vi "Host - TCP Serial.vi"(8 "error in (no error)":errorcluster, 9 "port":u16=4001, 10 "address":string="192.168.81.105") -> ()   [LabVIEW 2021]
panel:
  out "x-y":u32
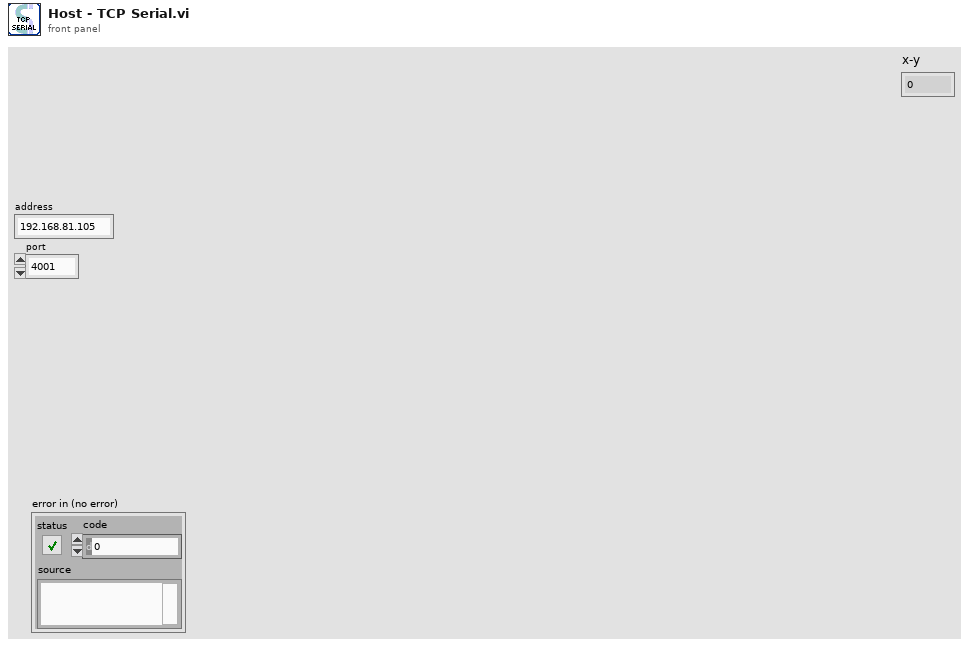
[diagram p1: front panel]
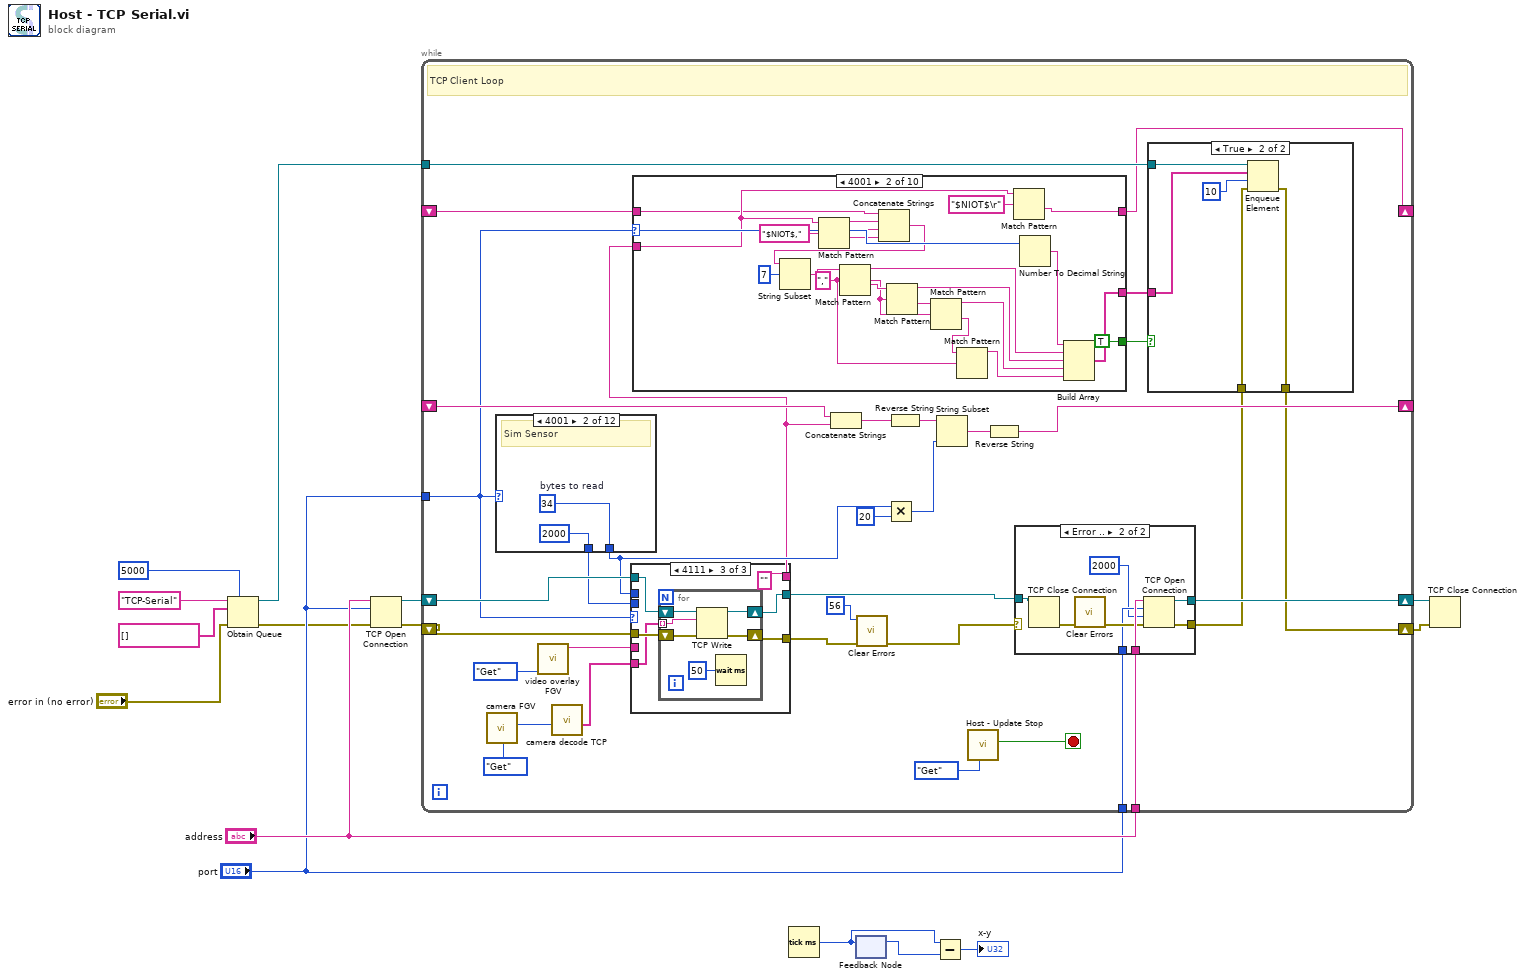
[diagram p0: block diagram]
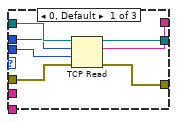
[diagram p3: hidden frame]
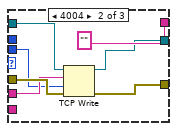
[diagram p4: hidden frame]
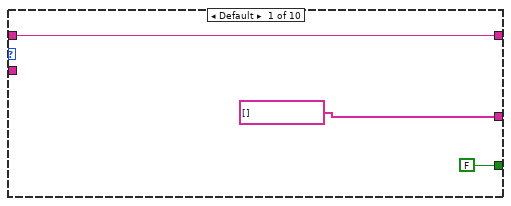
[diagram p5: hidden frame]
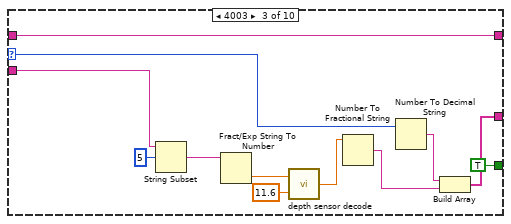
[diagram p6: hidden frame]
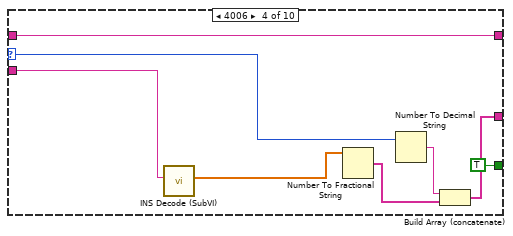
[diagram p7: hidden frame]
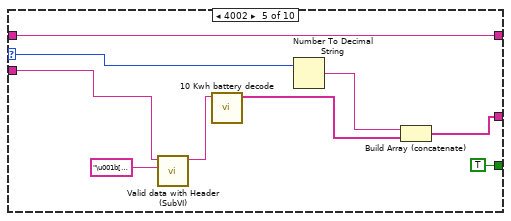
[diagram p8: hidden frame]
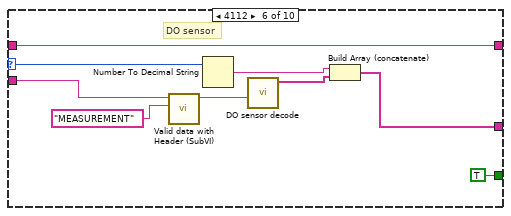
[diagram p9: hidden frame]
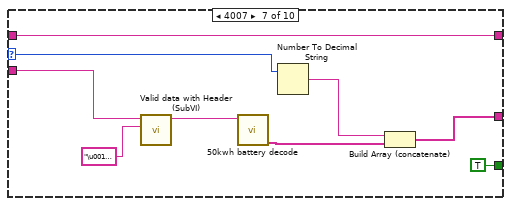
[diagram p10: hidden frame]
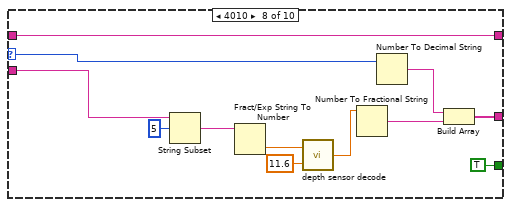
[diagram p11: hidden frame]
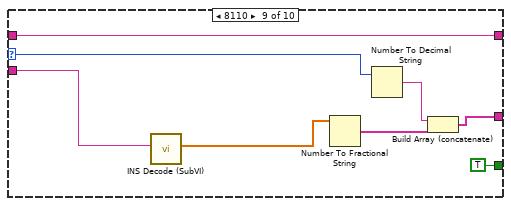
[diagram p12: hidden frame]
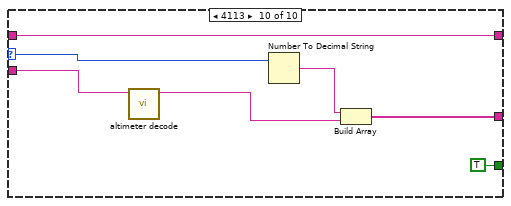
[diagram p13: hidden frame]
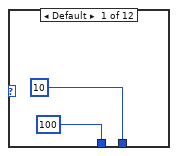
[diagram p15: hidden frame]
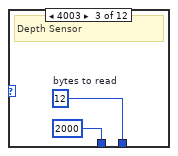
[diagram p16: hidden frame]
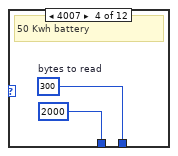
[diagram p17: hidden frame]
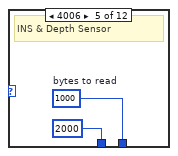
[diagram p18: hidden frame]
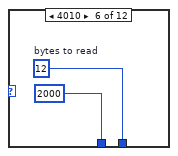
[diagram p19: hidden frame]
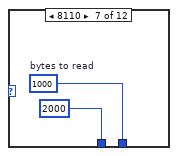
[diagram p20: hidden frame]
diagram:
  n1 = Obtain Queue(max queue size (-1, unlimited)=5000, name (unnamed)="TCP-Serial", element data type=string[] [], error in (no error)="error in (no error)") -> (queue out=w5:refnum<queue>, error out=w10:errorcluster)  [unwired: 1 in, 1 out]
  n2 = TCP Open Connection(address="address", remote port or service name="port", error in (no error)=w10) -> (connection ID=w15:refnum<k5>, error out=w14:errorcluster)  [unwired: 2 in]
  n3 = while {
    shift-right: [w41] -> _
    shift-left: _ -> [w44]
    tunnel: "port" -> [w25]
    tunnel: "address" -> [w33]
    tunnel: "port" -> [w32]
    tunnel: w5 -> [w30]
    shift-right: [w27] -> _
    shift-left: _ -> [w26]
    shift-right: [w34] -> w13
    shift-left: w15 -> [w48]
    shift-right: [w23] -> w1
    shift-left: w14 -> [w47]
    stop <- w37 stop-if-true
    # "TCP Client Loop"
    n4 = call "camera FGV.vi"("Operation"=enum16{"Init", "Get", "Set"}."Get") -> ("camera out"=w18:u32)  [unwired: 9 in, 1 out]
    n5 = case shown="4001" w25 {
      tunnel: [100 ("timeout ms (25000)") 2000 ("timeout ms (25000)") 2000 ("timeout ms (25000)") 2000 ("timeout ms (25000)") 2000 ("timeout ms (25000)") 2000 ("timeout ms (25000)") 2000 ("timeout ms (25000)") 2000 ("timeout ms (25000)") 2000 ("timeout ms (25000)") 2000 ("timeout ms (25000)") 0 ("timeout ms (25000)") 2000 ("timeout ms (25000)")] -> w46
      tunnel: [10 ("bytes to read") w194 w196 w198 w200 w202 w204 w206 22 ("bytes to read") 30 ("bytes to read") 0 ("bytes to read") 500 ("bytes to read")] -> w40
      frame Default {
      }
      frame 4001 {
        w194 = 34  # bytes to read
        # "Sim Sensor"
      }
      frame 4003 {
        w196 = 12  # bytes to read
        # "Depth Sensor"
      }
      frame 4007 {
        w198 = 300  # bytes to read
        # "50 Kwh battery"
      }
      frame 4006 {
        w200 = 1000  # bytes to read
        # "INS & Depth Sensor"
      }
      frame 4010 {
        w202 = 12  # bytes to read
      }
      frame 8110 {
        w204 = 1000  # bytes to read
      }
      frame 4002 {
        w206 = 1660  # bytes to read
        # "10kW battery"
      }
      frame 4113 {
        # "Altimeter"
      }
      frame 4004 {
      }
      frame 4111 {
      }
      frame 4112 {
        # "DO sensor"
      }
    }
    n6 = call "video overlay FGV.vi"("Operation"=enum16{"Init", "Get", "Set"}."Get") -> ("String"=w24:string)  [unwired: 10 in]
    n7 = call "camera decode TCP.vi"("Numeric"=w18) -> ("camera commands"=w17:string[])  [unwired: 10 in]
    n8 = case shown="4111" w25 {
      tunnel: [w62 w65 w74] -> w49
      tunnel: w48 -> [w61 w68 w73]
      tunnel: w47 -> [w60 w66 w72]
      tunnel: w46 -> [w59 w63 _]
      tunnel: w40 -> [w58 _ _]
      tunnel: [w57 w67 w75] -> w35
      tunnel: [w56 "" ("data out") "" ("data out")] -> w31
      tunnel: w24 -> [_ w64 _]
      tunnel: w17 -> [_ _ w71]
      frame 0, Default {
        n9 = TCP Read(connection ID=w61, bytes to read=w58, error in (no error)=w60, 9:w59) -> (connection ID out=w57:refnum<k5>, data out=w56:string, error out=w62:errorcluster)  [unwired: 1 in]
      }
      frame 4004 {
        n10 = TCP Write(connection ID=w68, data in=w64, error in (no error)=w66, 9:w63) -> (connection ID out=w67:refnum<k5>, error out=w65:errorcluster)  [unwired: 1 out]
      }
      frame 4111 {
        n11 = for {
          tunnel: w71 -> [w77] mode=indexing
          shift-right: [w81] -> w75
          shift-left: w73 -> [w79]
          shift-right: [w80] -> w74
          shift-left: w72 -> [w78]
          n12 = TCP Write(connection ID=w79, data in=w77, error in (no error)=w78) -> (connection ID out=w81:refnum<k5>, error out=w80:errorcluster)  [unwired: 1 in, 1 out]
          n13 = Wait (ms)(milliseconds to wait=u32 50) -> ()  [unwired: 1 out]
        }
      }
    }
    n14 = case shown="4001" w25 {
      selector: w25 -> [_ w105 w111 w125 w135 w140 w151 w165 w173 w179]
      tunnel: w31 -> [_ w88 w115 w122 w131 w144 w149 w157 w169 w180]
      tunnel: [string[] [] w106 w112 w126 w132 w137 w150 w163 w171 w178] -> w28
      tunnel: [w84 w89 w109 w123 w136 w145 w154 w166 w174 w181] -> w27
      tunnel: w26 -> [w84 w87 w109 w123 w136 w145 w154 w166 w174 w181]
      tunnel: [FALSE TRUE TRUE TRUE TRUE TRUE TRUE TRUE TRUE TRUE] -> w20
      frame Default {
      }
      frame 4001 {
        w96 = "," ("regular expression")
        n15 = Match Pattern(string=w88, regular expression="$NIOT$,") -> (before substring=w86:string, match substring=w93:string, after substring=w92:string)  [unwired: 1 in, 1 out]
        n16 = Concatenate Strings(w87, w86, w93, w92) -> (w91:string)
        n17 = String Subset(string=w91, offset (0)=7) -> (substring=w103:string)  [unwired: 1 out]
        n18 = Match Pattern(string=w103, regular expression=w96) -> (before substring=w100:string, after substring=w102:string)  [unwired: 1 in, 2 out]
        n19 = Match Pattern(string=w102, regular expression=w96) -> (before substring=w99:string, after substring=w101:string)  [unwired: 1 in, 2 out]
        n20 = Match Pattern(string=w101, regular expression=w96) -> (before substring=w98:string, after substring=w97:string)  [unwired: 1 in, 2 out]
        n21 = Match Pattern(string=w97, regular expression=w96) -> (before substring=w95:string)  [unwired: 1 in, 3 out]
        n22 = Match Pattern(string=w88, regular expression="$NIOT$\r") -> (after substring=w89:string)  [unwired: 1 in, 3 out]
        n23 = Number To Decimal String(number=w105) -> (decimal integer string=w104:string)  [unwired: 1 in]
        n24 = Build Array(w104, w100, w99, w98, w95) -> (w106:string[])
      }
      frame 4003 {
        n25 = String Subset(string=w115, offset (0)=5) -> (substring=w118:string)  [unwired: 1 out]
        n26 = Fract/Exp String To Number(string=w118) -> (number=w119:dbl)  [unwired: 4 out]
        n27 = call "depth sensor decode.vi"("Depth Offset"=11.6, "Input pressure"=w119) -> ("Depth in m"=w114:dbl)
        n28 = Number To Fractional String(number=w114) -> (F-format string=w113:string)  [unwired: 3 in]
        n29 = Number To Decimal String(number=w111) -> (decimal integer string=w110:string)  [unwired: 1 in]
        n30 = Build Array(w110, w113) -> (w112:string[])
      }
      frame 4006 {
        n31 = call "INS Decode (SubVI).vi"("read buffer"=w122) -> ("Data out"=w121:dbl[])  [unwired: 10 in]
        n32 = Number To Fractional String(number=w121) -> (F-format string=w127:string[])  [unwired: 3 in]
        n33 = Number To Decimal String(number=w125) -> (decimal integer string=w124:string)  [unwired: 1 in]
        n34 = Build Array (concatenate)(w124, w127) -> (w126:string[])
      }
      frame 4002 {
        n35 = call "Valid data with Header (SubVI).vi"("Header"="\u001b[2J\u001b[", "Input data"=w131) -> ("Valid Data"=w130:string)  [unwired: 9 in]
        n36 = call "10 Kwh battery decode.vi"("String"=w130) -> ("Battery Data"=w133:string[])  [unwired: 10 in]
        n37 = Number To Decimal String(number=w135) -> (decimal integer string=w134:string)  [unwired: 1 in]
        n38 = Build Array (concatenate)(w134, w133) -> (w132:string[])
      }
      frame 4112 {
        # "DO sensor"
        n39 = call "Valid data with Header (SubVI).vi"("Header"="MEASUREMENT", "Input data"=w144) -> ("Valid Data"=w142:string)  [unwired: 9 in]
        n40 = Number To Decimal String(number=w140) -> (decimal integer string=w139:string)  [unwired: 1 in]
        n41 = call "DO sensor decode.vi"("DO input"=w142) -> ("DO output string"=w138:string[])  [unwired: 9 in, 1 out]
        n42 = Build Array (concatenate)(w139, w138) -> (w137:string[])
      }
      frame 4007 {
        n43 = call "Valid data with Header (SubVI).vi"("Header"="\u0010\u0002", "Input data"=w149) -> ("Valid Data"=w148:string)  [unwired: 9 in]
        n44 = call "50kwh battery decode.vi"("data out"=w148) -> ("F-format string"=w152:string[])  [unwired: 9 in, 1 out]
        n45 = Number To Decimal String(number=w151) -> (decimal integer string=w153:string)  [unwired: 1 in]
        n46 = Build Array (concatenate)(w153, w152) -> (w150:string[])
      }
      frame 4010 {
        n47 = String Subset(string=w157, offset (0)=5) -> (substring=w161:string)  [unwired: 1 out]
        n48 = Fract/Exp String To Number(string=w161) -> (number=w162:dbl)  [unwired: 4 out]
        n49 = call "depth sensor decode.vi"("Depth Offset"=11.6, "Input pressure"=w162) -> ("Depth in m"=w158:dbl)
        n50 = Number To Fractional String(number=w158) -> (F-format string=w156:string)  [unwired: 3 in]
        n51 = Number To Decimal String(number=w165) -> (decimal integer string=w164:string)  [unwired: 1 in]
        n52 = Build Array(w164, w156) -> (w163:string[])
      }
      frame 8110 {
        n53 = call "INS Decode (SubVI).vi"("read buffer"=w169) -> ("Data out"=w170:dbl[])  [unwired: 10 in]
        n54 = Number To Fractional String(number=w170) -> (F-format string=w168:string[])  [unwired: 3 in]
        n55 = Number To Decimal String(number=w173) -> (decimal integer string=w172:string)  [unwired: 1 in]
        n56 = Build Array (concatenate)(w172, w168) -> (w171:string[])
      }
      frame 4113 {
        n57 = call "altimeter decode.vi"("string"=w180) -> ("before substring"=w176:string)  [unwired: 10 in]
        n58 = Number To Decimal String(number=w179) -> (decimal integer string=w177:string)  [unwired: 1 in]
        n59 = Build Array(w177, w176) -> (w178:string[])
      }
    }
    n60 = Concatenate Strings(w44, w31) -> (w45:string)
    n61 = call <vilib>:"Clear Errors.vi"("error in (no error)"=w49, "specific error code to clear (0: all)"=56) -> ("error out"=w36:errorcluster)  [unwired: 4 in, 1 out]
    n62 = Multiply(x=w40, y=20) -> (x*y=w38:i32)
    n63 = Reverse String(1:w45) -> (0:w42:string)
    n64 = String Subset(string=w42, length (rest)=w38) -> (substring=w43:string)  [unwired: 1 in]
    n65 = call "Host - Update Stop.vi"("Operation"=enum16{"Init", "Get", "Set"}."Get") -> ("Stop?"=w37:bool)  [unwired: 9 in, 1 out]
    n66 = Reverse String(1:w43) -> (0:w41:string)
    n67 = case shown="Error .." w36 {
      selector: w36 -> [w183 _]
      tunnel: [w183 w191] -> w29
      tunnel: w35 -> [w182 w189]
      tunnel: [w182 w188] -> w34
      tunnel: w33 -> [_ w187]
      tunnel: w32 -> [_ w185]
      frame No Error {
      }
      frame Error {
        n68 = TCP Close Connection(connection ID=w189) -> (error out=w190:errorcluster)  [unwired: 2 in, 1 out]
        n69 = call <vilib>:"Clear Errors.vi"("error in (no error)"=w190) -> ("error out"=w186:errorcluster)  [unwired: 5 in, 1 out]
        n70 = TCP Open Connection(address=w187, remote port or service name=w185, timeout ms (60000)=2000, error in (no error)=w186) -> (connection ID=w188:refnum<k5>, error out=w191:errorcluster)  [unwired: 1 in]
      }
    }
    n71 = case shown="True" w20 {
      tunnel: w30 -> [_ w55]
      tunnel: w29 -> [w50 w54]
      tunnel: w28 -> [_ w53]
      tunnel: [w50 w51] -> w23
      frame False {
      }
      frame True {
        n72 = Enqueue Element(queue=w55, element=w53, timeout in ms (-1)=10, error in (no error)=w54) -> (error out=w51:errorcluster)  [unwired: 2 out]
      }
    }
  }
  n73 = Tick Count (ms)() -> (millisecond timer value=w3:u32)
  n74 = feedback-in #1(w3) -> ()
  n75 = feedback #1() -> (w4:u32)  [unwired: 1 in]
  n76 = Subtract(x=w3, y=w4) -> (x-y=→"x-y":u32)
  n77 = TCP Close Connection(connection ID=w13, error in (no error)=w1) -> ()  [unwired: 1 in, 2 out]
